vi "GENERACION_REPORTE_CON_-PARAMETROS.vi"() -> ()   [LabVIEW 2021]
uses:
  <vilib>/Utility/NIReport.llb/Report Type.ctl
  <vilib>/Utility/NIReport.llb/Append Report Text (str wrap).vi
  <vilib>/Utility/NIReport.llb/NI_report.lvclass
  <vilib>/Utility/NIReport.llb/NI_ReportGenerationCore.lvlib
panel:
  in  "template (empty)":path
  in  "Array":cluster{"Class":string, string, string}[](array[cluster])=[{"Class"="Rojo Cola", "298.000000", "Aprobado"}, {"Class"="Rojo Cola", "298.000000", "Aprobado"}]
  in  "direccion para guardar":path
  out "new picture":picture
  in  "path to JPEG file":path
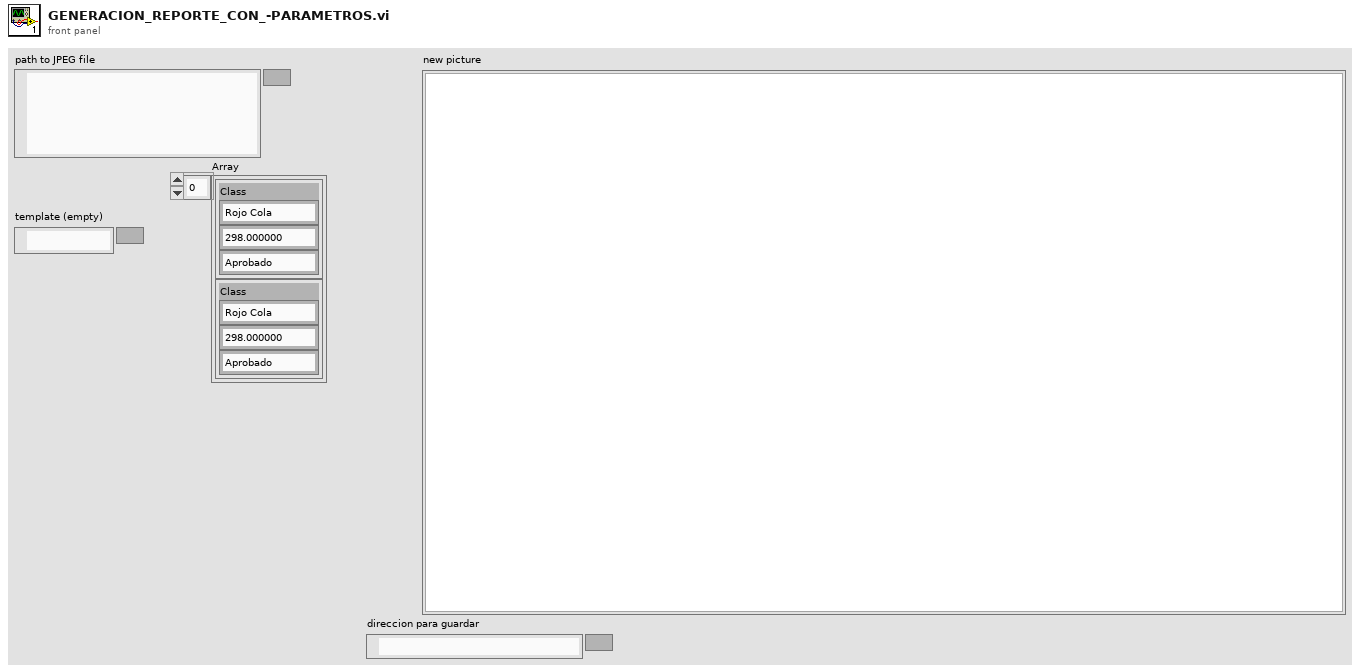
[diagram p1: front panel]
types:
  T1 = typedef "NI_ReportGenerationCore.lvlib/Report Type.ctl" = enum16{"HTML", "Word", "Excel"}
  T2 = cluster{"Charset (-1)":i16, "Weight (-1)":i16, "Name":string, "Size":string}
  T3 = cluster{"Italic":enum16{"Italic Unchanged", "Italic On", "Italic Off"}, "Strike Through":enum16{"Strike Through Unchanged", "Strike Through On", "Strike Through Off"}, "Underline":enum16{"Underline Unchanged", "Underline On", "Underline Off"}, "Bold":enum16{"Bold Unchanged", "Bold On", "Bold Off"}}
  T4 = typedef "imagedata.ctl" = cluster{"image type":i32, "image depth":i32, "image":u8[], "mask":u8[], "colors":u32[], "Rectangle":cluster{"left":i16, "top":i16, "right":i16, "bottom":i16}}
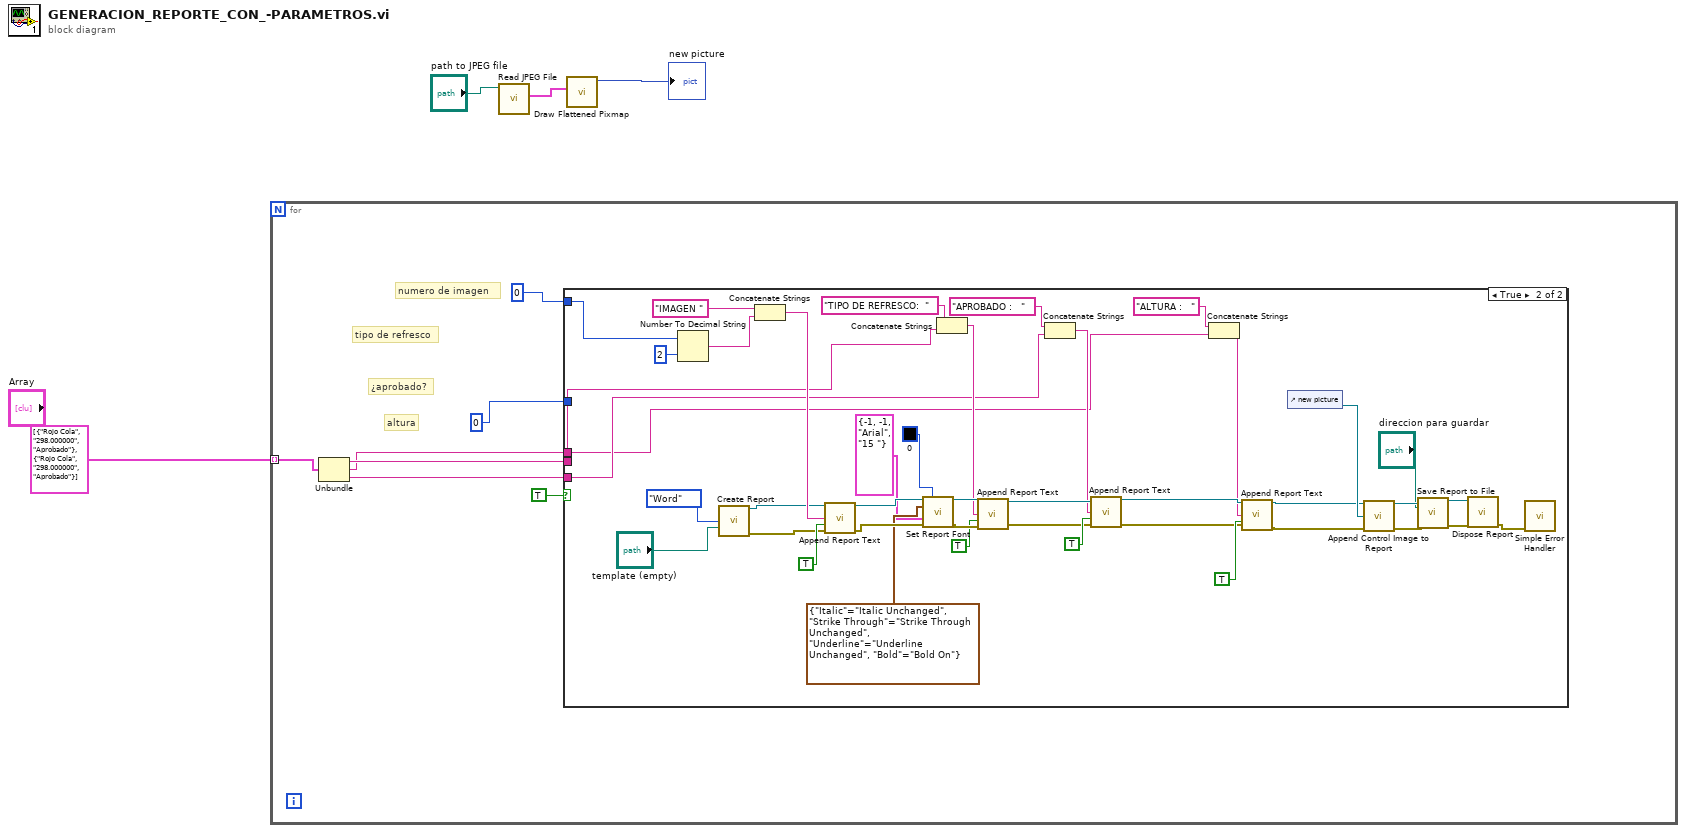
[diagram p0: block diagram]
diagram:
  n1 = for {
    tunnel: cluster{"Class":string, string, string}[] [{"Class"="Rojo Cola", "298.000000", "Aprobado"}, {"Class"="Rojo Cola", "298.000000", "Aprobado"}] ("Array") -> [w8] mode=indexing
    # "altura"
    # "¿aprobado?"
    # "tipo de refresco"
    # "numero de imagen"
    n2 = Unbundle(w8) -> ("Class"=w7:string, w5:string, w6:string)
    n3 = case shown="True" TRUE {
      tunnel: 0 -> [_ w38]
      tunnel: 0 -> [_ _]
      tunnel: w7 -> [_ w18]
      tunnel: w6 -> [_ w17]
      tunnel: w5 -> [_ w16]
      frame False {
      }
      frame True {
        n4 = Number To Decimal String(number=w38, width (-)=i16 2) -> (decimal integer string=w37:string)
        n5 = call <vilib>:"Create Report.vi"("report type"=Report_Type."Word", "template (empty)"="template (empty)") -> ("report out"=w15:refnum<class "NI_report.lvclass">, "error out"=w14:errorcluster)  [unwired: 12 in]
        n6 = Concatenate Strings("IMAGEN " ("text"), w37) -> (w36:string)
        n7 = call-poly <vilib>:"Append Report Text.vi"("report in"=w15, "text"=w36, "append on new line? (F)"=TRUE, "error in (no error)"=w14) -> ("report out"=w48:refnum<class "NI_report.lvclass">, "error out"=w47:errorcluster)  [unwired: 8 in, 2 out]
        n8 = call-dynamic "Set Report Font.vi"("report in"=w48, "text color (unchanged)"=u32 0, "text options"=T3 {"Italic"=enum."Italic Unchanged", "Strike Through"=enum."Strike Through Unchanged", "Underline"=enum."Underline Unchanged", "Bold"=enum."Bold On"}, "font settings"=T2 {"Charset (-1)"=-1, "Weight (-1)"=-1, "Name"="Arial", "Size"="15 "}, "error in (no error)"=w47) -> ("report out"=w35:refnum<class "NI_report.lvclass">, "error out"=w34:errorcluster)  [unwired: 8 in, 1 out]
        n9 = Concatenate Strings("TIPO DE REFRESCO:  " ("text"), w18) -> (w31:string)
        n10 = call-poly <vilib>:"Append Report Text.vi"("report in"=w35, "text"=w31, "append on new line? (F)"=TRUE, "error in (no error)"=w34) -> ("report out"=w26:refnum<class "NI_report.lvclass">, "error out"=w21:errorcluster)  [unwired: 8 in, 2 out]
        n11 = Concatenate Strings("APROBADO :   " ("text"), w17) -> (w20:string)
        n12 = call-poly <vilib>:"Append Report Text.vi"("report in"=w26, "text"=w20, "append on new line? (F)"=TRUE, "error in (no error)"=w21) -> ("report out"=w25:refnum<class "NI_report.lvclass">, "error out"=w22:errorcluster)  [unwired: 8 in, 2 out]
        n13 = Concatenate Strings("ALTURA :   " ("text"), w16) -> (w19:string)
        n14 = call-poly <vilib>:"Append Report Text.vi"("report in"=w25, "text"=w19, "append on new line? (F)"=TRUE, "error in (no error)"=w22) -> ("report out"=w24:refnum<class "NI_report.lvclass">, "error out"=w23:errorcluster)  [unwired: 8 in, 2 out]
        n15 = control-ref of="new picture"() -> (w43:refnum<vi>)
        n16 = call-dynamic "Append Control Image to Report.vi"("report in"=w24, "ctrl reference"=w43, "error in (no error)"=w23) -> ("report out"=w53:refnum<class "NI_report.lvclass">, "error out"=w52:errorcluster)  [unwired: 9 in, 2 out]
        n17 = call-dynamic "Save Report to File.vi"("report in"=w53, "report file path"="direccion para guardar", "error in (no error)"=w52) -> ("report out"=w51:refnum<class "NI_report.lvclass">, "error out"=w50:errorcluster)  [unwired: 11 in]
        n18 = call-dynamic "Dispose Report.vi"("report in"=w51, "error in (no error)"=w50) -> ("error out"=w42:errorcluster)  [unwired: 13 in]
        n19 = call <vilib>:"Simple Error Handler.vi"("error in (no error)"=w42) -> ()  [unwired: 4 in, 5 out]
      }
    }
  }
  n20 = call <vilib>:"Read JPEG File.vi"("path to JPEG file"="path to JPEG file") -> ("image data"=w3:T4)  [unwired: 8 in, 2 out]
  n21 = call <vilib>:"Draw Flattened Pixmap.vi"("image data"=w3) -> ("new picture"=→"new picture":picture)  [unwired: 8 in]
